vi "IsModeEnables.vi"(8 "error in (no error)":errorcluster, 10 "Mode value":string, 11 "ModeCol in":refnum<class "ModeCol.lvclass">) -> (0 "error out":errorcluster, 2 "Disable / Enable":bool caption="Enable?", 3 "ModeCol out":refnum<class "ModeCol.lvclass">)   [LabVIEW 2013, in "ModeCol.lvclass"]
uses:
  ModeCol.lvclass
  ModeCol.lvclass/ModeCol.ctl
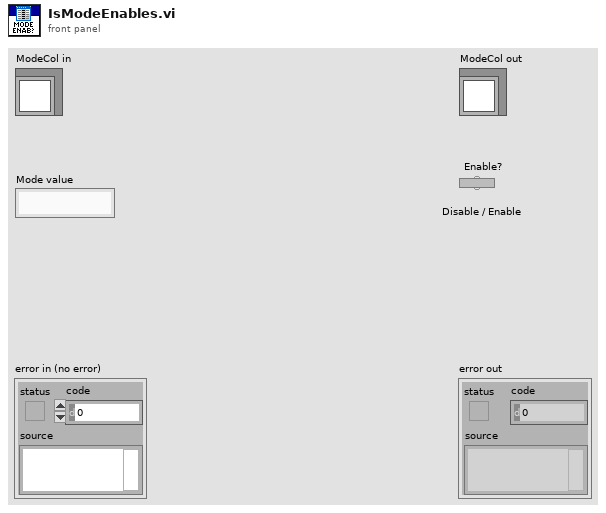
[diagram p1: front panel]
types:
  T1 = cluster{"Mode":string, "ModeTag":string, "Disables?":bool}[]
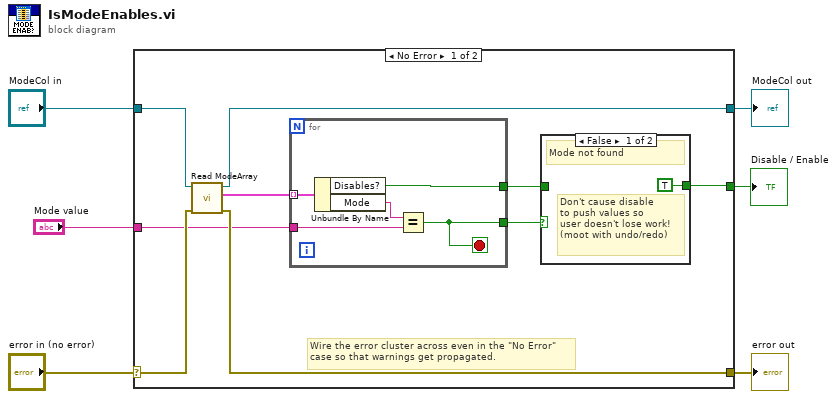
[diagram p0: block diagram]
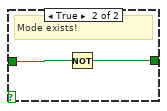
[diagram p2: hidden frame]
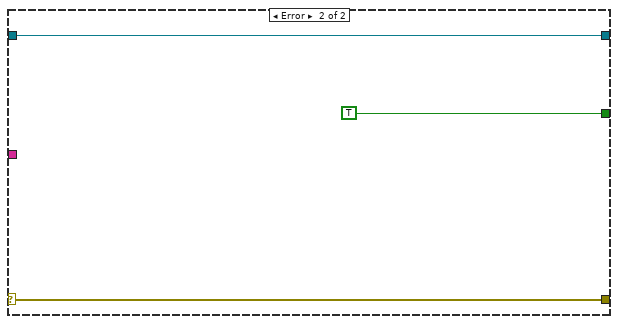
[diagram p3: hidden frame]
diagram:
  n1 = case shown="No Error" "error in (no error)" {
    selector: "error in (no error)" -> [w13 w26]
    tunnel: [w11 w26] -> w5
    tunnel: [w14 w25] -> w3
    tunnel: "ModeCol in" -> [w15 w25]
    tunnel: "Mode value" -> [w10 _]
    tunnel: [w7 TRUE] -> w2
    frame No Error {
      # "Wire the error cluster across even in the \"No Error\"\ncase so that warnings get propagated."
      n2 = call "Read ModeArray.vi"("error in (no error)"=w13, "ModeCol in"=w15) -> ("error out"=w11:errorcluster, "Array"=w12:T1, "ModeCol out"=w14:refnum<class "ModeCol.lvclass">)  [unwired: 7 in]
      n3 = for {
        tunnel: w12 -> [w23] mode=indexing
        tunnel: w10 -> [w21]
        tunnel: [w19] -> w8
        tunnel: [w20] -> w9
        stop <- w20 stop-if-true
        n4 = Unbundle By Name(w23) -> ("Disables?"=w19:bool, "Mode"=w22:string)
        n5 = Equal?(x=w22, y=w21) -> (x = y?=w20:bool)
      }
      n6 = case shown="False" w9 {
        tunnel: w8 -> [_ w18]
        tunnel: [TRUE w17] -> w7
        frame False {
          # "Don't cause disable\nto push values so \nuser doesn't lose work!\n(moot with undo/redo)"
          # "Mode not found"
        }
        frame True {
          # "Mode exists!"
          n7 = Not(x=w18) -> (.not. x?=w17:bool)
        }
      }
    }
    frame Error {
    }
  }
  "error out" <- w5
  "ModeCol out" <- w3
  "Disable / Enable" <- w2
